vi "niRFUtil WFM Normalize Waveform.vi"(7 "Waveform In":T2 {"y" format="%.2f"; "dx" format="%^.2e"; "x0" format="%^.2e"}, 13 "Burst Present":T1) -> (8 "Waveform Out":T2 {"y" format="%.2f"; "dx" format="%^.2e"; "x0" format="%^.2e"})   [LabVIEW 2015, in "niRFUtil.lvlib"]
doc: "(c) Copyright 2006, National Instruments, Inc. This VI may not be duplicated, sold, or distributed without written consent from National Instruments."
uses:
  niRFUtil.lvlib
  Includes/niRFUtil INC Complex Waveform.ctl
  Includes/niRFUtil INC Complex Array.ctl
  Includes/niRFUtil INC Burst Present.ctl
  Includes/niRFUtil INC Edge Detection Settings.ctl
  Includes/niRFUtil INC Edge Type.ctl
  niRFUtil WFM Concatenate Waveforms (complex wfm).vi
  niRFUtil WFM Parse Waveform - Duration (complex wfm).vi
  niRFUtil WFM Detect Multiple Bursts (complex wfm).vi
  niRFUtil WFM Detect Edge (complex wfm).vi
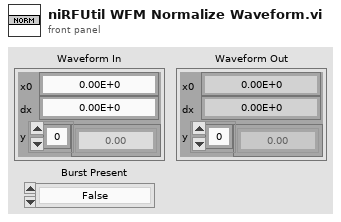
[diagram p1: front panel]
types:
  T1 = typedef "niRFUtil.lvlib/niRFUtil INC Burst Present.ctl" = enum16{"False", "True", "Multiple Bursts"}
  T2 = typedef "niRFUtil.lvlib/niRFUtil INC Complex Waveform.ctl" = cluster{"x0":dbl, "dx":dbl, "y":T3}
  T3 = typedef "niRFUtil.lvlib/niRFUtil INC Complex Array.ctl" = csg[]
  T4 = typedef "niRFUtil.lvlib/niRFUtil INC Edge Detection Settings.ctl" = cluster{"Mode":enum16{"Sliding Window", "Threshold"}, "Sliding Window Settings":cluster{"Chunks":i32, "Threshold (dB)":dbl}, "Threshold Settings":cluster{"Threshold Level (dB)":dbl, "Minimum Quiet Time (s)":dbl, "Threshold Type":enum16{"Relative", "Absolute"}}}
  T5 = typedef "niRFUtil.lvlib/niRFUtil INC Edge Type.ctl" = enum16{"Rising", "Falling"}
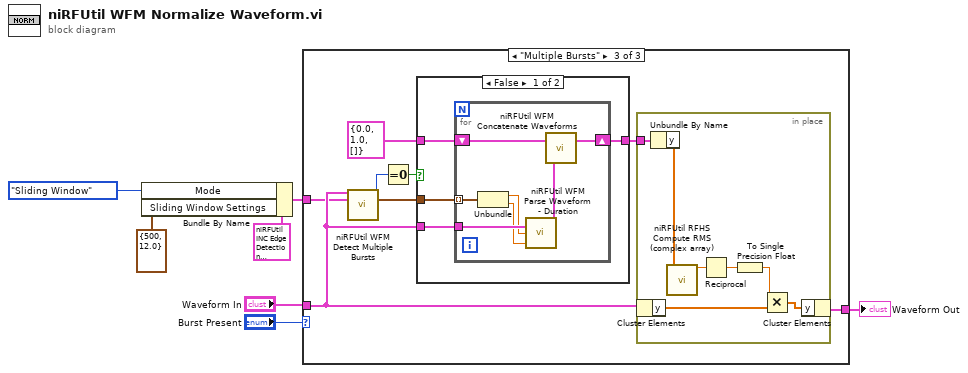
[diagram p0: block diagram]
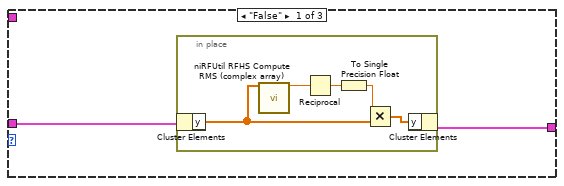
[diagram p2: hidden frame]
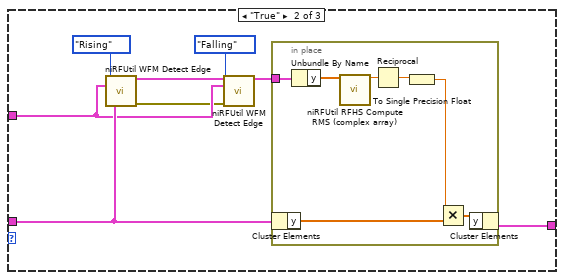
[diagram p3: hidden frame]
diagram:
  n1 = Bundle By Name(cluster=T4 {"Mode"=enum."Sliding Window", "Sliding Window Settings"={"Chunks"=500, "Threshold (dB)"=12.0}, "Threshold Settings"={"Threshold Level (dB)"=-50.0, "Minimum Quiet Time (s)"=0.0001, "Threshold Type"=enum."Absolute"}} ("Burst Detection Settings"), "Mode"=enum16{"Sliding Window", "Threshold"}."Sliding Window", "Sliding Window Settings"=cluster{"Chunks":i32, "Threshold (dB)":dbl} {"Chunks"=500, "Threshold (dB)"=12.0}) -> (w1:T4)
  n2 = case shown="\"Multiple Bursts\"" "Burst Present" {
    tunnel: "Waveform In" -> [w9 w22 w35]
    tunnel: [w8 w21 w37] -> w5
    tunnel: w1 -> [_ w17 w31]
    frame "False" {
      n3 = in-place {
        n4 = in-place-cluster #1(w9) -> ("y"=w11:T3)
        n5 = call "niRFUtil RFHS Compute RMS (complex array).vi"("Complex Array (V)"=w11) -> ("RMS (V)"=w10:sgl)  [unwired: 14 in]
        n6 = Reciprocal(x=w10) -> (1/x=w14:sgl)
        n7 = To Single Precision Float(number=w14) -> (single precision float=w13:sgl)
        n8 = Multiply(x=w13, y=w11) -> (x*y=w12:T3)
        n9 = in-place-cluster #1("y"=w12) -> (w8:T2)
      }
    }
    frame "True" {
      n10 = call-poly "niRFUtil WFM Detect Edge.vi"("Input Waveform"=w22, "Edge Detection Settings"=w17, "Edge Type"=niRFUtil_INC_Edge_Type."Rising") -> ("Output Waveform"=w19:T2, "error out"=w16:errorcluster)  [unwired: 9 in, 2 out]
      n11 = call-poly "niRFUtil WFM Detect Edge.vi"("Input Waveform"=w19, "Edge Detection Settings"=w17, "Edge Type"=niRFUtil_INC_Edge_Type."Falling", "error in (no error)"=w16) -> ("Output Waveform"=w15:T2)  [unwired: 8 in, 3 out]
      n12 = in-place {
        in-place-border: w15 -> [w25]
        n13 = in-place-cluster #2(w22) -> ("y"=w29:T3)
        n14 = Unbundle By Name(w25) -> ("y"=w24:T3)
        n15 = call "niRFUtil RFHS Compute RMS (complex array).vi"("Complex Array (V)"=w24) -> ("RMS (V)"=w23:sgl)  [unwired: 14 in]
        n16 = Reciprocal(x=w23) -> (1/x=w27:sgl)
        n17 = To Single Precision Float(number=w27) -> (single precision float=w26:sgl)
        n18 = Multiply(x=w26, y=w29) -> (x*y=w28:T3)
        n19 = in-place-cluster #2("y"=w28) -> (w21:T2)
      }
    }
    frame "Multiple Bursts" {
      n20 = call-poly "niRFUtil WFM Detect Multiple Bursts.vi"("Waveform In (Ohm Voltage)"=w35, "Burst Detection Settings"=w31) -> ("Number of Bursts Detected"=w32:i32, "Burst Positions"=w36:cluster{"Start (s)":dbl, "Duration (s)":dbl}[])  [unwired: 12 in]
      n21 = Equal To 0?(x=w32) -> (x = 0?=w33:bool)
      n22 = case shown="False" w33 {
        tunnel: w36 -> [w41 _]
        tunnel: w35 -> [w40 w49]
        tunnel: [w39 w49] -> w34
        tunnel: T2 {"x0"=0.0, "dx"=1.0, "y"=[]} ("Waveform Constant") -> [w38 _]
        frame False {
          n23 = for {
            tunnel: w41 -> [w47] mode=indexing
            tunnel: w40 -> [w48]
            shift-right: [w42] -> w39
            shift-left: w38 -> [w44]
            n24 = Unbundle(w47) -> ("Start (s)"=w46:dbl, "Duration (s)"=w45:dbl)
            n25 = call-poly "niRFUtil WFM Parse Waveform - Duration.vi"("Duration (Inf)"=w45, "Start (-Inf)"=w46, "Waveform In"=w48) -> ("Waveform Out"=w43:T2)  [unwired: 2 in]
            n26 = call-poly "niRFUtil WFM Concatenate Waveforms.vi"("Waveform 2 In"=w43, "Waveform 1 In"=w44) -> ("Waveform Out"=w42:T2)  [unwired: 1 in]
          }
        }
        frame True {
        }
      }
      n27 = in-place {
        in-place-border: w34 -> [w52]
        n28 = in-place-cluster #3(w35) -> ("y"=w56:T3)
        n29 = Unbundle By Name(w52) -> ("y"=w51:T3)
        n30 = call "niRFUtil RFHS Compute RMS (complex array).vi"("Complex Array (V)"=w51) -> ("RMS (V)"=w50:sgl)  [unwired: 14 in]
        n31 = Reciprocal(x=w50) -> (1/x=w54:sgl)
        n32 = To Single Precision Float(number=w54) -> (single precision float=w53:sgl)
        n33 = Multiply(x=w53, y=w56) -> (x*y=w55:T3)
        n34 = in-place-cluster #3("y"=w55) -> (w37:T2)
      }
    }
  }
  "Waveform Out" <- w5
